vi "setUp.vi"(8 "error in (no error)":errorcluster, 11 "reference in":refnum<class "TestCSMSuite.lvclass">) -> (0 "error out":errorcluster, 3 "reference out":refnum<class "TestCSMSuite.lvclass">)   [LabVIEW 2017, in "TestCSMSuite.lvclass"]
doc: "setUp runs prior to the test method during test execution. Use this method to initialize any object data required by your tests."
uses:
  TestCSMSuite.lvclass
  C:/Program Files (x86)/National Instruments/LabVIEW 2017/vi.lib/addons/_JKI Toolkits/VI Tester/TestSuite.llb/TestSuite.lvclass
  src/user.lib/_NEVSTOP/Communicable State Machine(CSM)/addons/Logger/CSM File Logger Limit.ctl
  TestCSMSuite.lvclass/TestCSMSuite.ctl
  src/user.lib/_NEVSTOP/Communicable State Machine(CSM)/_Support/GlobalEvent/GEvt-Convert Filter Rules - Periodic Setting Only.vi
  src/user.lib/_NEVSTOP/Communicable State Machine(CSM)/_Support/GlobalEvent/LogFilter/SettingVIs/Set Periodic Log Filter.vi
  src/user.lib/_NEVSTOP/Communicable State Machine(CSM)/_Support/GlobalEvent/LogFilter/LogFilter.lvclass
  <vilib>/addons/_JKI Toolkits/VI Tester/TestSuite.llb/TestSuite.lvclass
  CSM/CSM-Testcase.lvlib
  src/user.lib/_NEVSTOP/Communicable State Machine(CSM)/addons/Logger/CSM File Logger.lvlib
  src/user.lib/_NEVSTOP/Communicable State Machine(CSM)/Communicable State Machine.lvlib
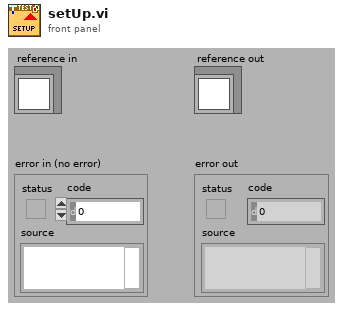
[diagram p1: front panel]
types:
  T1 = typedef "CSM File Logger.lvlib/CSM File Logger Limit.ctl" = cluster{"file size (in bytes)":i64, "file num":i32}
  T2 = cluster{"Enable":bool, "Threshold(#/s)":dbl, "CheckPeriod(s)":dbl}
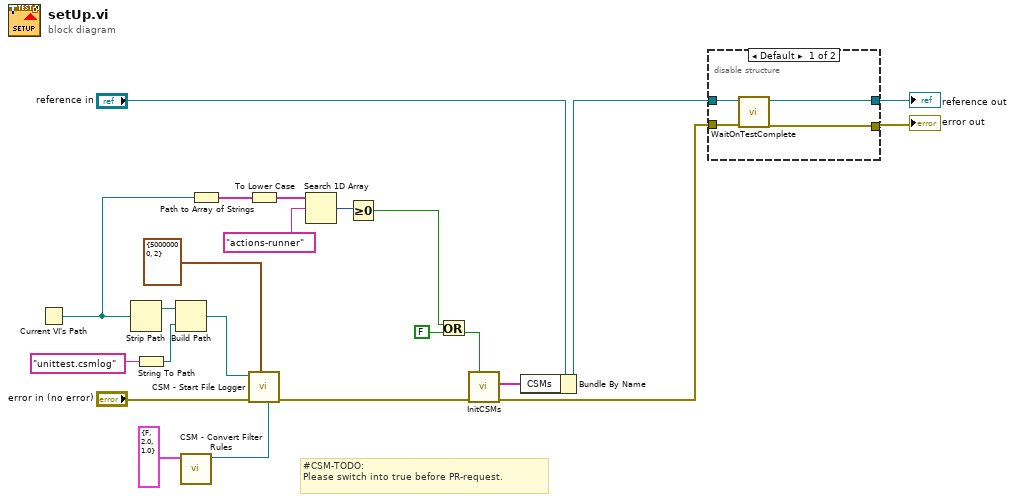
[diagram p0: block diagram]
diagram:
  # "#CSM-TODO:\nPlease switch into true before PR-request."
  n1 = Current VI's Path() -> (path=w6:path)
  n2 = Strip Path(path=w6) -> (stripped path=w15:path)  [unwired: 1 out]
  n3 = String To Path(string="unittest.csmlog") -> (path=w16:path)
  n4 = Build Path(base path=w15, name or relative path=w16) -> (appended path=w14:path)
  n5 = call-poly "CSM - Convert Filter Rules.vi"("PeriodicMessageFilter"=T2 {"Enable"=FALSE, "Threshold(#/s)"=2.0, "CheckPeriod(s)"=1.0}) -> ("GlobalLogFilter"=w10:refnum<class "LogFilter.lvclass">)  [unwired: 10 in]
  n6 = Path to Array of Strings(0:w6) -> (2:w5:string[])  [unwired: 1 out]
  n7 = To Lower Case(string=w5) -> (all lower case string=w3:string[])
  n8 = call "CSM - Start File Logger.vi"("Filter Rules"=w10, "Log Limit"=T1 {"file size (in bytes)"=50000000, "file num"=2}, "Error In"="error in (no error)", "Log File Path"=w14) -> ("error out"=w18:errorcluster)  [unwired: 5 in, 2 out]
  n9 = Search 1D Array(1D array=w3, element="actions-runner") -> (index of element=w2:i32)  [unwired: 1 in]
  n10 = Greater Or Equal To 0?(x=w2) -> (x >= 0?=w1:bool)
  n11 = Or(x=w1, y=FALSE ("Enable Conditional Building lvlibp?")) -> (x .or. y?=w7:bool)
  n12 = call "InitCSMs.vi"("Enable Conditional Building lvlibp?"=w7, "error in"=w18) -> ("error out"=w21:errorcluster, "CSMs"=w11:string[])  [unwired: 8 in]
  n13 = Bundle By Name(cluster="reference in", "CSMs"=w11) -> (w12:refnum<class "TestCSMSuite.lvclass">)
  n14 = disable-structure shown="Default" {
    disable-tunnel: w12 -> [w27 w28]
    disable-tunnel: [w26 w28] -> w23
    disable-tunnel: w21 -> [w25 w29]
    disable-tunnel: [w24 w29] -> w22
    frame condition #0 (active) {
      n15 = call <vilib>:"WaitOnTestComplete.vi"("error in (no error)"=w25, "TestSuite in"=w27) -> ("error out"=w24:errorcluster, "TestSuite out"=w26:refnum<class "TestCSMSuite.lvclass">)  [unwired: 8 in]
    }
    frame condition #1 {
    }
  }
  "error out" <- w22
  "reference out" <- w23
